vi "Update_Path.vi"(7 "new path":path, 8 "error in (no error)":errorcluster, 9 "destTag":string, 10 "destinations in":refnum<class "IB_Destination.lvclass">[](array[class]), 11 "IB_DestTree in":refnum<class "IB_Tree_Dest.lvclass">) -> (0 "error out":errorcluster, 1 "duplicate?":bool, 2 "destinations out":refnum<class "IB_Destination.lvclass">[](array[class]), 3 "IB_DestTree out":refnum<class "IB_Tree_Dest.lvclass">, 5 "edits":T1[](array[typedef]))   [LabVIEW 2020, in "IB_Tree_Dest.lvclass"]
uses:
  <vilib>/AppBuilder/IB_Classes/Tree_Dest/IB_Tree_Dest.lvclass
  <vilib>/AppBuilder/IB_Classes/Tree_Dest/IB_Tree_Dest.lvclass/IB_Tree_Dest.ctl
  <vilib>/AppBuilder/IB_Classes/Destination/IB_Destination.lvclass
  <vilib>/AppBuilder/IB_Classes/Tree_Dest/destEdits_operation.ctl
  <vilib>/AppBuilder/IB_Classes/Tree_Dest/destEdits_edit.ctl
  <vilib>/AppBuilder/IB_Classes/Tree_Dest/destEdits_rename.ctl
  <vilib>/AppBuilder/IB_Classes/Destination/absFolder/absFolder.lvclass
  <vilib>/AppBuilder/IB_Classes/Tree/IB_Tree.lvclass
  e:/builds/penguin/labview/branches/2020/dev/dist/vi.lib/AppBuilder/IB_Classes/Tree/IB_Tree.lvclass
  e:/builds/penguin/labview/branches/2020/dev/dist/vi.lib/AppBuilder/IB_Classes/Tree_Dest/IB_Tree_Dest.lvclass
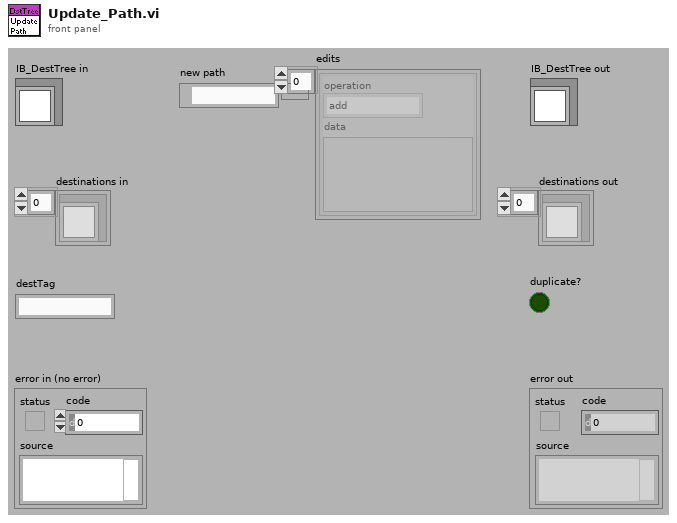
[diagram p1: front panel]
types:
  T1 = typedef "destEdits_edit.ctl" = cluster{"operation":T2, "data":variant}
  T2 = typedef "destEdits_operation.ctl" = enum16{"add", "remove", "rename", "sort children", "default dir changed"}
  T3 = typedef "destEdits_rename.ctl" = cluster{"child tag":string, "left cell string":string}
  T4 = typedef "IB_Destination.ctl" = cluster{"name":string, "unlock":bool, "parentTag":string, "destTag":string, "eng_installPath":string}
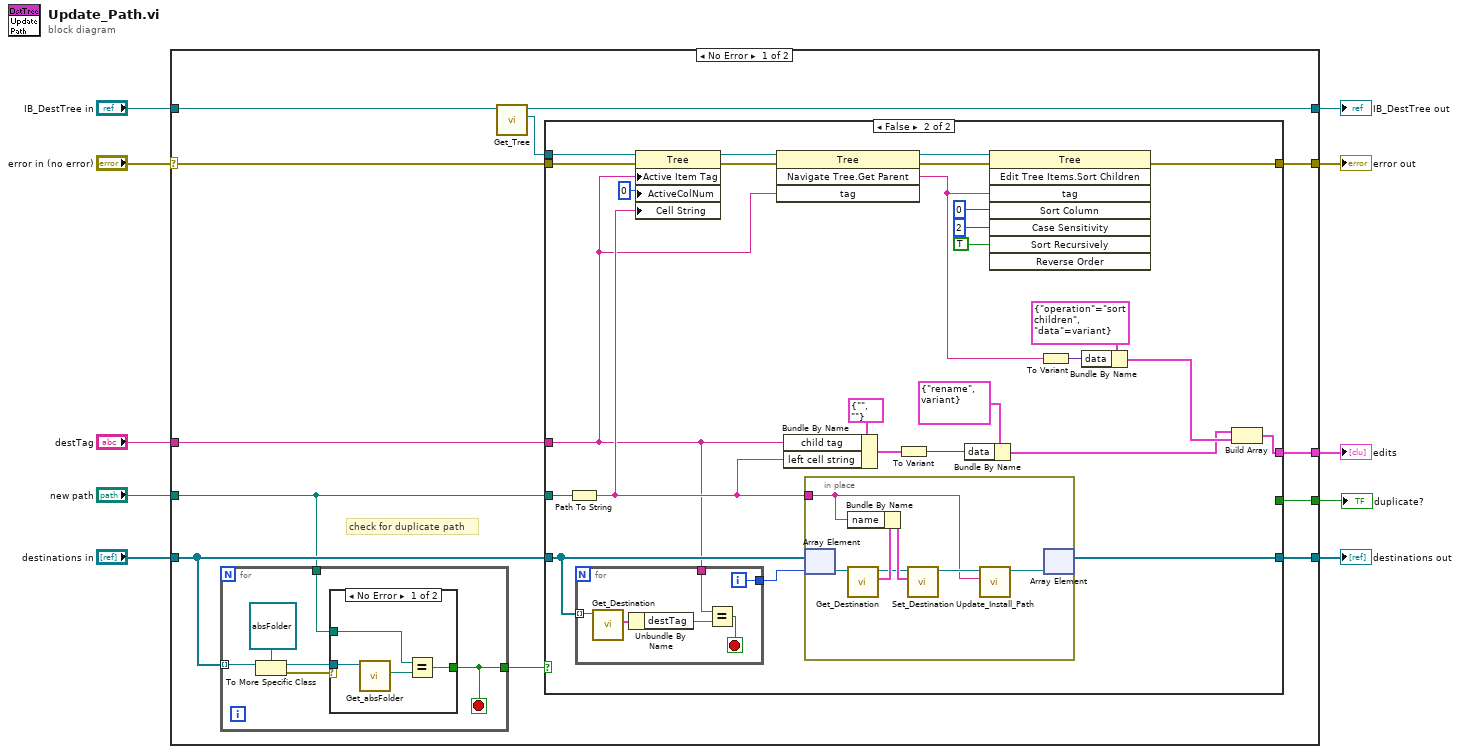
[diagram p0: block diagram]
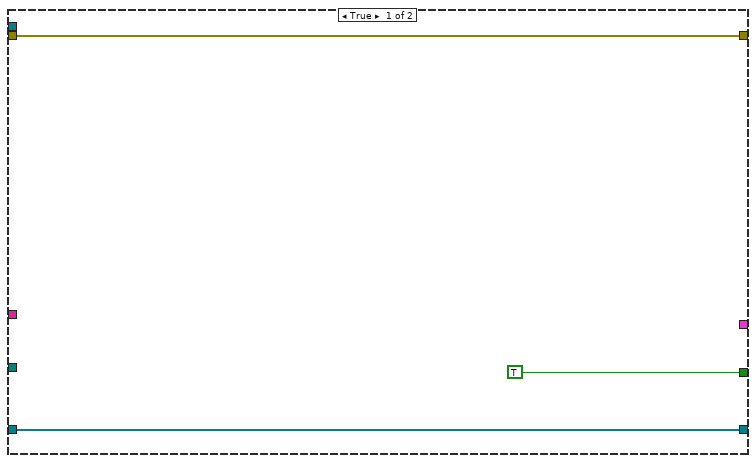
[diagram p3: hidden frame]
diagram:
  n1 = case shown="No Error" "error in (no error)" {
    selector: "error in (no error)" -> [w14 w78]
    tunnel: [w22 w78] -> w9
    tunnel: [w11 w77] -> w7
    tunnel: "IB_DestTree in" -> [w12 w77]
    tunnel: "destTag" -> [w21 _]
    tunnel: "new path" -> [w16 _]
    tunnel: "destinations in" -> [w17 w76]
    tunnel: [w20 _] -> w3
    tunnel: [w19 w76] -> w2
    tunnel: [w18 _] -> w1
    frame No Error {
      # "check for duplicate path"
      n2 = for {
        tunnel: w17 -> [w28] mode=indexing
        tunnel: w16 -> [w24]
        tunnel: [w23] -> w15
        stop <- w23 stop-if-true
        n3 = To More Specific Class(target class=refnum<class "absFolder.lvclass"> refnum ("absFolder in"), reference=w28) -> (specific class reference=w26:refnum<class "absFolder.lvclass">, error out=w25:errorcluster)  [unwired: 1 in]
        n4 = case shown="No Error" w25 {
          tunnel: w26 -> [w32 _]
          tunnel: w24 -> [w30 _]
          tunnel: [w29 _] -> w23
          frame No Error {
            n5 = call <vilib>:"Get_absFolder.vi"("absFolder in"=w32) -> ("Path"=w31:path)  [unwired: 1 in, 9 out]
            n6 = Equal?(x=w30, y=w31) -> (x = y?=w29:bool)
          }
          frame Error {
          }
        }
      }
      n7 = call <vilib>:"Get_Tree.vi"("IB_Tree in"=w12) -> ("ctl"=w13:refnum<vi>, "IB_Tree out"=w11:refnum<class "IB_Tree_Dest.lvclass">)  [unwired: 1 in, 8 out]
      n8 = case shown="False" w15 {
        tunnel: [w35 w40] -> w22
        tunnel: w14 -> [w35 w61]
        tunnel: w13 -> [_ w60]
        tunnel: w21 -> [_ w39]
        tunnel: w16 -> [_ w52]
        tunnel: w17 -> [w34 w59]
        tunnel: [_ w36] -> w20
        tunnel: [w34 w58] -> w19
        tunnel: [TRUE _] -> w18
        frame True {
        }
        frame False {
          n9 = Path To String(path=w52) -> (string=w51:string)
          n10 = for {
            tunnel: w59 -> [w75] mode=indexing
            tunnel: w39 -> [w72]
            tunnel: [w70] -> w53
            i -> [w70]
            stop <- w71 stop-if-true
            n11 = call <vilib>:"Get_Destination.vi"("IB_Destination in"=w75) -> ("data"=w74:T4)  [unwired: 1 in, 9 out]
            n12 = Unbundle By Name(w74) -> ("destTag"=w73:string)
            n13 = Equal?(x=w72, y=w73) -> (x = y?=w71:bool)
          }
          n14 = property class="Tree"(reference=w60, error in=w61, "Active Item Tag"=w39, "ActiveColNum"=0 ("Active Cell:Active Column Number"), "Cell String"=w51) -> (reference out=w42:refnum<vi>, error out=w41:errorcluster)
          n15 = invoke class="Tree" method="Navigate Tree.Get Parent"(reference=w42, error in=w41, "tag"=w39) -> (reference out=w48:refnum<vi>, error out=w49:errorcluster, "Navigate Tree:Get Parent"=w43:string)  [unwired: 1 in, 1 out]
          n16 = Bundle By Name(cluster=T3 {"child tag"="", "left cell string"=""} ("rename"), "child tag"=w39, "left cell string"=w51) -> (w57:T3)
          n17 = in-place {
            in-place-border: w51 -> [w63]
            n18 = in-place-array #1(w59, w53) -> (w66:refnum<class "IB_Destination.lvclass">)
            n19 = call <vilib>:"Get_Destination.vi"("IB_Destination in"=w66) -> ("data"=w68:T4, "IB_Destination out"=w67:refnum<class "IB_Destination.lvclass">)  [unwired: 1 in, 8 out]
            n20 = Bundle By Name(cluster=w68, "name"=w63) -> (w69:T4)
            n21 = call <vilib>:"Set_Destination.vi"("data"=w69, "IB_Destination in"=w67) -> ("IB_Destination out"=w65:refnum<class "IB_Destination.lvclass">)  [unwired: 1 in, 8 out]
            n22 = call-dynamic "Update_Install_Path.vi"("destName"=w63, "IB_Destination in"=w65) -> ("IB_Destination out"=w64:refnum<class "IB_Destination.lvclass">)  [unwired: 1 in, 8 out]
            n23 = in-place-array #1(w64) -> (w58:refnum<class "IB_Destination.lvclass">[])  [unwired: 1 out]
          }
          n24 = To Variant(anything=w57) -> (Variant=w56:variant)
          n25 = Bundle By Name(cluster=T1 {"operation"=enum."rename", "data"=variant} ("edit"), "data"=w56) -> (w37:T1)
          n26 = invoke class="Tree" method="Edit Tree Items.Sort Children"(reference=w48, error in=w49, "tag"=w43, "Sort Column"=0, "Case Sensitivity"=2, "Sort Recursively"=TRUE ("Carry Children?")) -> (error out=w40:errorcluster)  [unwired: 2 in, 7 out]
          n27 = To Variant(anything=w43) -> (Variant=w44:variant)
          n28 = Bundle By Name(cluster=T1 {"operation"=enum."sort children", "data"=variant} ("edit"), "data"=w44) -> (w38:T1)
          n29 = Build Array(w37, w38) -> (w36:T1[])
        }
      }
    }
    frame Error {
    }
  }
  "error out" <- w9
  "IB_DestTree out" <- w7
  "edits" <- w3
  "destinations out" <- w2
  "duplicate?" <- w1
